vi "Draw Lines at Point.vi"(4 "GraphBGK":u32(colorbox), 6 "color(black)":u32(colorbox), 7 "pixel center":cluster{"horizontal":i16, "vertical":i16}, 9 "Vertical Line?":bool, 10 "Horizontal Line?":bool, 11 "new picture in":picture) -> (3 "new picture out":picture)   [LabVIEW 2014, in "Graph Extensions.lvlib"]
uses:
  Graph Extensions.lvlib
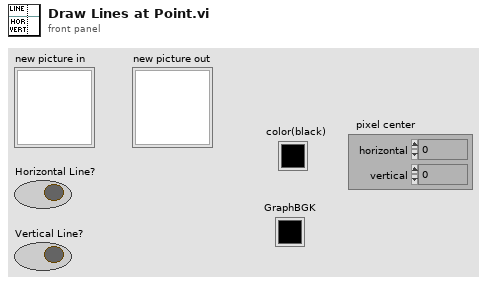
[diagram p1: front panel]
types:
  T1 = cluster{"Width":u16, "Style":enum32{"Solid", "Dash", "Dot", "DashDot", "DashDotDot"}}
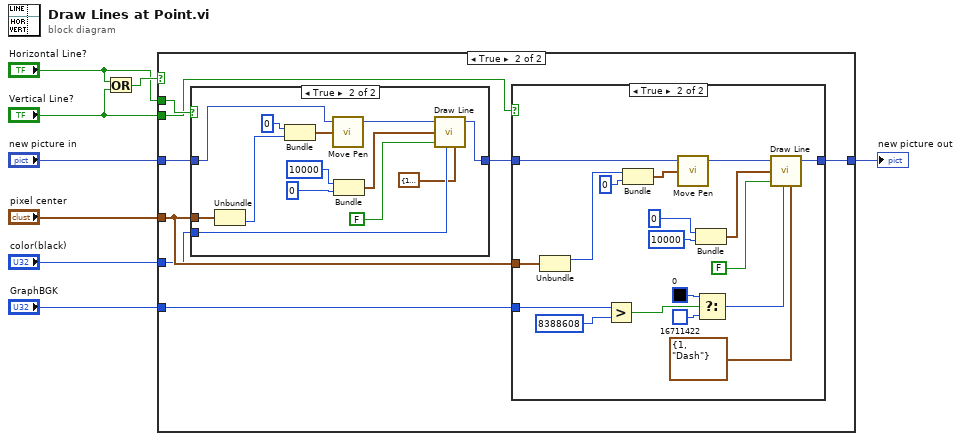
[diagram p0: block diagram]
diagram:
  n1 = Or(x="Horizontal Line?", y="Vertical Line?") -> (x .or. y?=w3:bool)
  n2 = case shown="True" w3 {
    tunnel: "Vertical Line?" -> [_ w14]
    tunnel: "new picture in" -> [w9 w17]
    tunnel: [w9 w11] -> w8
    tunnel: "color(black)" -> [_ w12]
    tunnel: "pixel center" -> [_ w13]
    tunnel: "Horizontal Line?" -> [_ w16]
    tunnel: "GraphBGK" -> [_ w10]
    frame False {
    }
    frame True {
      n3 = case shown="True" w16 {
        tunnel: w17 -> [w37 w43]
        tunnel: [w37 w42] -> w15
        tunnel: w12 -> [_ w41]
        tunnel: w13 -> [_ w40]
        frame False {
        }
        frame True {
          n4 = Unbundle(w40) -> ("vertical"=w39:i16)  [unwired: 1 out]
          n5 = Bundle(i16 0, "vertical"=w39) -> (w46:cluster{i16, "vertical":i16})  [unwired: 1 in]
          n6 = call <vilib>:"Move Pen.vi"("new position"=w46, "picture"=w43) -> ("new picture"=w44:picture)  [unwired: 3 in]
          n7 = Bundle(i16 10000, i16 0) -> (w48:cluster{i16, i16})  [unwired: 1 in]
          n8 = call <vilib>:"Draw Line.vi"("picture"=w44, "end point"=w48, "absolute coordinates?(T)"=FALSE, "color(black)"=w41, "pen"=T1 {"Width"=1, "Style"=enum."Dot"}) -> ("new picture"=w42:picture)  [unwired: 4 in]
        }
      }
      n9 = case shown="True" w14 {
        tunnel: [w18 w30] -> w11
        tunnel: w13 -> [_ w29]
        tunnel: w15 -> [w18 w27]
        tunnel: w10 -> [_ w23]
        frame False {
        }
        frame True {
          n10 = Unbundle(w29) -> ("horizontal"=w26:i16)  [unwired: 1 out]
          n11 = Greater?(x=w23, y=u32 8388608) -> (0:w22:bool)
          n12 = Bundle("horizontal"=w26, i16 0) -> (w32:cluster{"horizontal":i16, i16})  [unwired: 1 in]
          n13 = call <vilib>:"Move Pen.vi"("new position"=w32, "picture"=w27) -> ("new picture"=w31:picture)  [unwired: 3 in]
          n14 = Bundle(i16 0, i16 10000) -> (w34:cluster{i16, i16})  [unwired: 1 in]
          n15 = Select(t=u32 0, s=w22, f=u32 16711422) -> (s? t:f=w19:u32)
          n16 = call <vilib>:"Draw Line.vi"("picture"=w31, "end point"=w34, "absolute coordinates?(T)"=FALSE, "color(black)"=w19, "pen"=T1 {"Width"=1, "Style"=enum."Dash"}) -> ("new picture"=w30:picture)  [unwired: 4 in]
        }
      }
    }
  }
  "new picture out" <- w8
